vi "FPGA_1.vi"() -> ()   [LabVIEW 2019]
uses:
  <vilib>/rvi/Emulation/niFpgaGetClockAttributes.vi
  <vilib>/rvi/Emulation/niFpgaSctlEmulationGetInTimedLoop.vi
  <vilib>/rvi/Emulation/niFpgaEmulationReportErrorSimple.vi
  <vilib>/rvi/eio/common/nirviEmuTemplateMethod_errors.vi
  <vilib>/rvi/DataTransferAndStorage/Container/Common/niFpgaContainerExecOnDevCompGetState.vi
  <vilib>/rvi/Emulation/niFpgaEmulationIsFPGAContextNoSignature.vi
  <vilib>/rvi/errors/niFpgaSetErrorForExecOnDevCompSimple.vi
  <vilib>/rvi/eio/common/nirviEmuReportErrorAndStop.vi
  <vilib>/rvi/DataTransferAndStorage/Container/Common/niFpgaContainerGetUniqueNameForEmu.vi
  <vilib>/rvi/FIFO/Fifo_Resource/nirvififoEmulationSetSize.vi
  <vilib>/rvi/FIFO/Fifo_Resource/nirviFifoEmulationQueueMgr.vi
  <instcachedir>/0/nirviFifoEmulationQueueMgr_E5CAEC123FF24DC58D834DCA3CDAA9B5.lvgen/nirviFifoEmulationQueueMgr_E5CAEC123FF24DC58D834DCA3CDAA9B5_003.vi
  <vilib>/rvi/FIFO/Fifo_Resource/nirvififoEmulationDetermineInputValidOut.vi
  <vilib>/rvi/FIFO/Fifo_Resource/nirvififoEmulationCreateLock.vi
  <vilib>/rvi/Emulation/niFpgaProcessEmulError.vi
  <vilib>/rvi/FIFO/Fifo_Resource/nirvififoEmulationObtainLock.vi
  <vilib>/rvi/FIFO/Fifo_Resource/nirvififoEmulationReleaseLock.vi
  <vilib>/rvi/occurrence/nirviWaitOnOccurrenceBase.vi
  <vilib>/rvi/errors/nirviReportUnexpectedCaseInternalError.vi
  <vilib>/rvi/errors/nirviReportUnexpectedCaseInternalError (U32).vi
  <vilib>/Utility/error.llb/Clear Errors.vi
  <vilib>/rvi/interface/RandomDataEmulation/niFpgaRandomDataHandleErrors.vi
  <vilib>/rvi/Emulation/niFpgaCriticalErrorInLSC.vi
  <vilib>/eio/EIONode/EIONode.xnode
  <vilib>/rvi/DataTransferAndStorage/Container/XNode/niFpgaContainer.xnode
  <vilib>/rvi/FIFO/Fifo_Resource/niFpgaFifoEmulationRefIn.vi
panel:
  out "AI1":i16(graph)
  out "AI1":i16
  out "AI0":i16
  out "AI0":i16(graph)
  in  "stop":bool
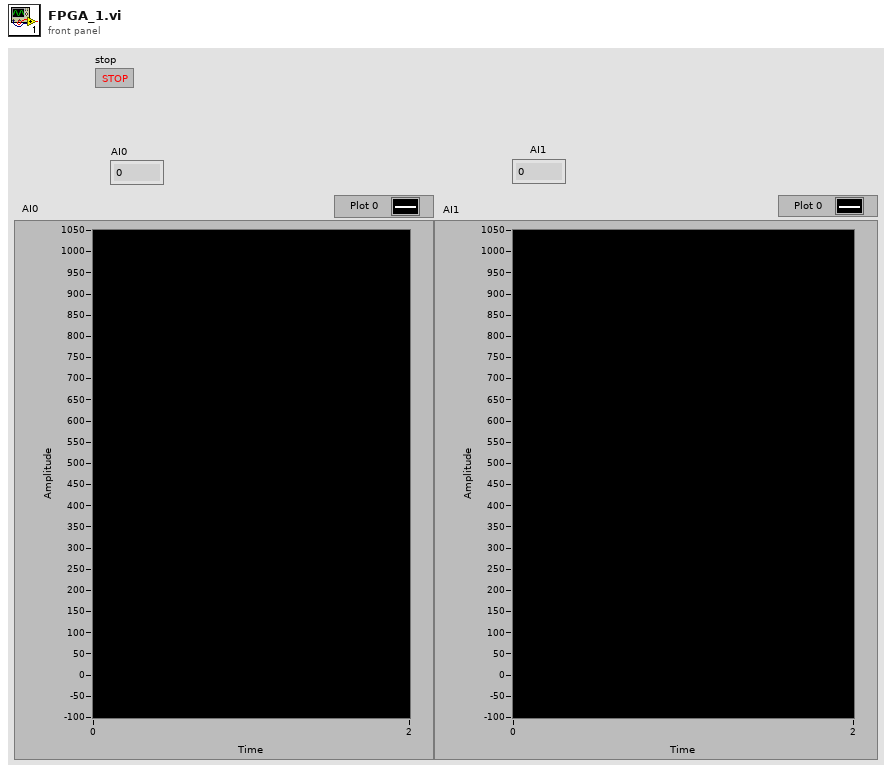
[diagram p1: front panel]
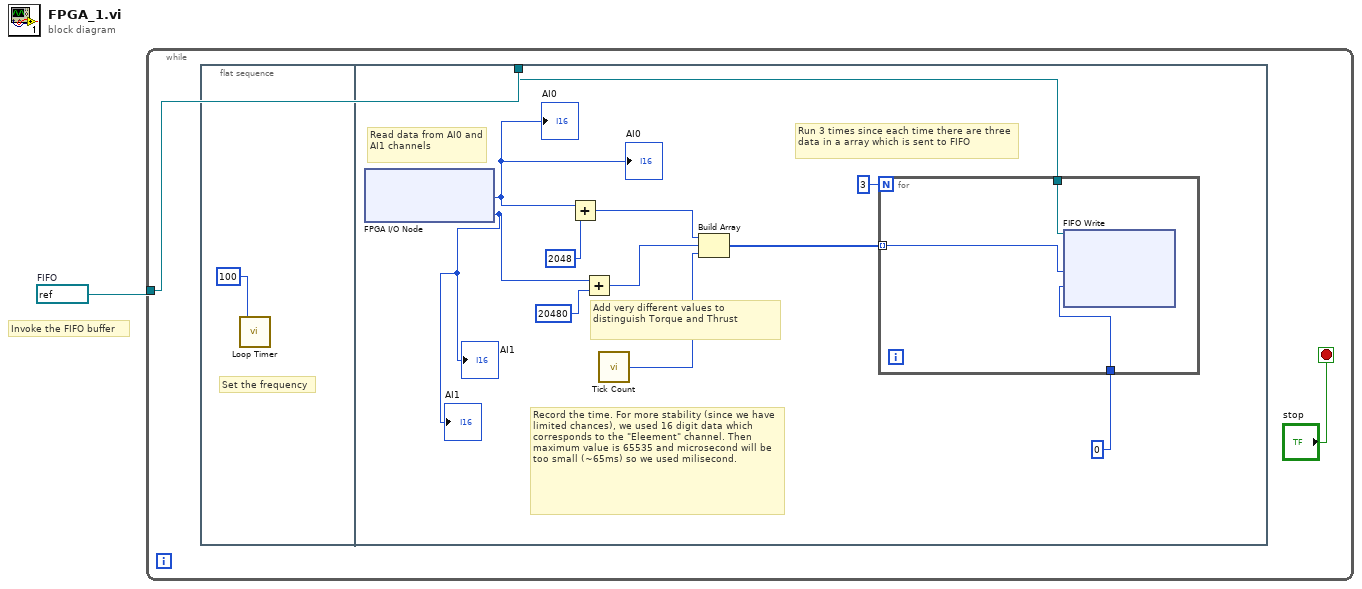
[diagram p0: block diagram]
diagram:
  w1 = refnum<k21> "FIFO"  # FIFO
  # "Invoke the FIFO buffer"
  n1 = while {
    tunnel: w1 -> [w2]
    stop <- "stop" stop-if-true
    n2 = flat-sequence {
      tunnel: w2 -> [w15]
      frame #0 {
        # "Set the frequency"
        n3 = call "Loop Timer"("Count(uSec)"=u32 100) -> ()  [unwired: 1 out]
      }
      frame #1 {
        # "Read data from AI0 and AI1 channels"
        # "Run 3 times since each time there are three data in a array which is sent to FIFO"
        # "Add very different values to distinguish Torque and Thrust"
        # "Record the time. For more stability (since we have limited chances), we used 16 digit data which corresponds to the \"Eleement\" channel. Then maximum value is 65535 and microsecond will be too small (~65ms) so we used milisecond."
        n4 = xnode "FPGA I/O Node"() -> ("ConnectorC/AI0"=w13:i16, "ConnectorC/AI1"=w8:i16)  [unwired: 2 in, 2 out]
        "AI0" <- w13
        "AI0" <- w13
        "AI1" <- w8
        "AI1" <- w8
        n5 = Add(x=w13, y=i16 2048) -> (x+y=w11:i16)
        n6 = Add(x=w8, y=i16 20480) -> (x+y=w12:i16)
        n7 = call "Tick Count"() -> ("Tick Count(mSec)"=w7:u16)
        n8 = Build Array(w11, w12, w7) -> (w9:u16[])
        n9 = for {
          N: 3 -> [_]
          tunnel: w15 -> [w18]
          tunnel: 0 ("Timeout") -> [w17]
          tunnel: w9 -> [w16] mode=indexing
          n10 = xnode ("FIFO Write")("Element"=w16, "Timeout"=w17, "FIFO In"=w18) -> ()  [unwired: 2 out]
        }
      }
    }
  }
